vi "LeCroy Wave Series Acquire Multiple Waveforms.vi"() -> ()   [LabVIEW 2018]
doc: "This example shows how to configure multiple channels and acquire waveforms from multiple channels."
uses:
  Public/Data/Read Multiple Waveforms.vi
  LeCroy Wave Series.lvlib
panel:
  in  "Channel (1: Channel 2)":u16(ring)=1 items=["Channel 1", "Channel 2", "Channel 3", "Channel 4"]
  in  "Channel (0: Channel 1)":u16(ring) items=["Channel 1", "Channel 2", "Channel 3", "Channel 4"]
  in  "Vertical Coupling (0: A1M)":u16(ring) items=["A1M", "D1M", "D50", "Ground"]
  in  "Vertical Coupling (0: A1M)":u16(ring) items=["A1M", "D1M", "D50", "Ground"]
  in  "Vertical Offset (0.0 V)":dbl
  in  "Vertical Offset (0.0 V)":dbl
  in  "Probe Attenuation (-1)":dbl=-1.0
  in  "Probe Attenuation (-1)":dbl=-1.0
  in  "Timeout (10000 ms)":u32=10000
  out "Waveform Data":waveform(dbl)[](graph)
  in  "VISA resource name":refnum<visa-resource-name>
  # "(c) 2005 - 2012 NATIONAL INSTRUMENTS.  ALL RIGHTS RESERVED."
  # "Channel A"
  # "Channel B"
  # "Note:\nThis VI will time out without acquiring any data if the input signal on channel 1 does not cross 0 V trigger level with positive slope.\nFor more details on triggering pleas see the Edge Triggered Acquisition Example VI."
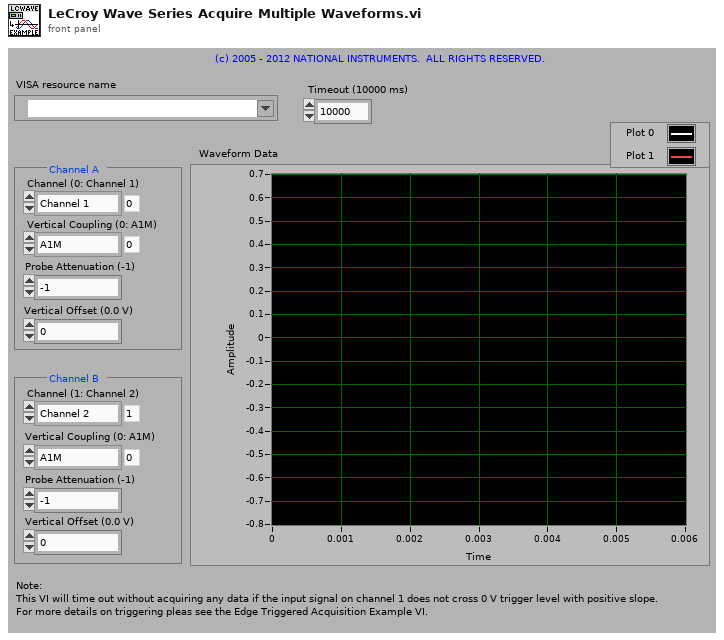
[diagram p1: front panel]
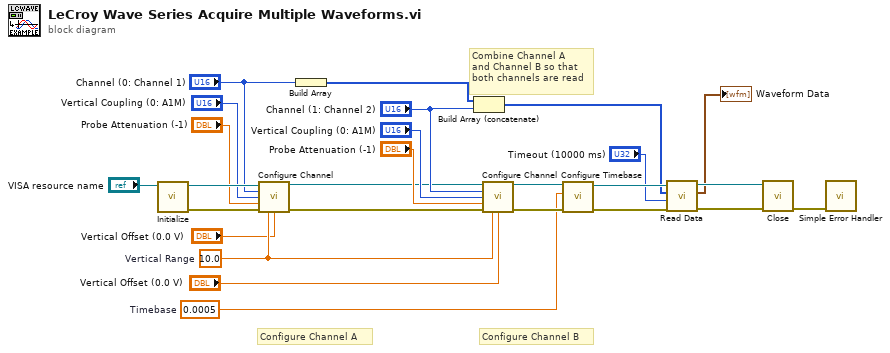
[diagram p0: block diagram]
diagram:
  w14 = 10.0  # Vertical Range
  w13 = 0.0005  # Timebase
  # "Combine Channel A\nand Channel B so that\nboth channels are read"
  # "Configure Channel B"
  # "Configure Channel A"
  n1 = call "Initialize.vi"("VISA resource name"="VISA resource name") -> ("error out"=w21:errorcluster, "VISA resource name out"=w22:refnum<visa-resource-name>)  [unwired: 9 in]
  n2 = call "Configure Channel.vi"("VISA resource name"=w22, "Channel (0: Channel 1)"="Channel (0: Channel 1)", "Vertical Coupling (0: A1M)"="Vertical Coupling (0: A1M)", "Probe Attenuation (-1.0)"="Probe Attenuation (-1)", "error in (no error)"=w21, "Vertical Range (10.0 V)"=w14, "Vertical Offset (0.0 V)"="Vertical Offset (0.0 V)") -> ("VISA resource name out"=w3:refnum<visa-resource-name>, "error out"=w2:errorcluster)  [unwired: 7 in]
  n3 = Build Array("Channel (0: Channel 1)") -> (w5:u16[])
  n4 = Build Array (concatenate)(w5, "Channel (1: Channel 2)") -> (w4:u16[])
  n5 = call "Configure Channel.vi"("VISA resource name"=w3, "Channel (0: Channel 1)"="Channel (1: Channel 2)", "Vertical Coupling (0: A1M)"="Vertical Coupling (0: A1M)", "Probe Attenuation (-1.0)"="Probe Attenuation (-1)", "error in (no error)"=w2, "Vertical Range (10.0 V)"=w14, "Vertical Offset (0.0 V)"="Vertical Offset (0.0 V)") -> ("VISA resource name out"=w20:refnum<visa-resource-name>, "error out"=w19:errorcluster)  [unwired: 7 in]
  n6 = call "Configure Timebase.vi"("error in (no error)"=w19, "Timebase (0.0005 s)"=w13, "VISA resource name"=w20) -> ("error out"=w17:errorcluster, "VISA resource name out"=w18:refnum<visa-resource-name>)  [unwired: 7 in]
  n7 = call-poly "Read Data.vi"("error in (no error)"=w17, "Timeout (10000 ms)"="Timeout (10000 ms)", "Channels"=w4, "VISA resource name"=w18) -> ("error out"=w23:errorcluster, "Waveform Data"=→"Waveform Data":waveform(dbl)[], "VISA resource name out"=w24:refnum<visa-resource-name>)  [unwired: 5 in]
  n8 = call "Close.vi"("error in (no error)"=w23, "VISA resource name"=w24) -> ("error out"=w25:errorcluster)  [unwired: 9 in]
  n9 = call <vilib>:"Simple Error Handler.vi"("error in (no error)"=w25) -> ()  [unwired: 4 in, 5 out]
